vi "2401 Write Data.vi"(7 "I/V":bool, 8 "Compliance":dbl, 10 "Level (A/V)":dbl) -> (1 "Resistance":dbl format="%#_6e", 2 "Current":dbl format="%#_6e", 3 "Voltage":dbl format="%_6e")   [LabVIEW 2011]
panel:
  out "number 4":dbl format="%#_6e"
  out "number5":dbl format="%#_6e"
  out "read buffer":string
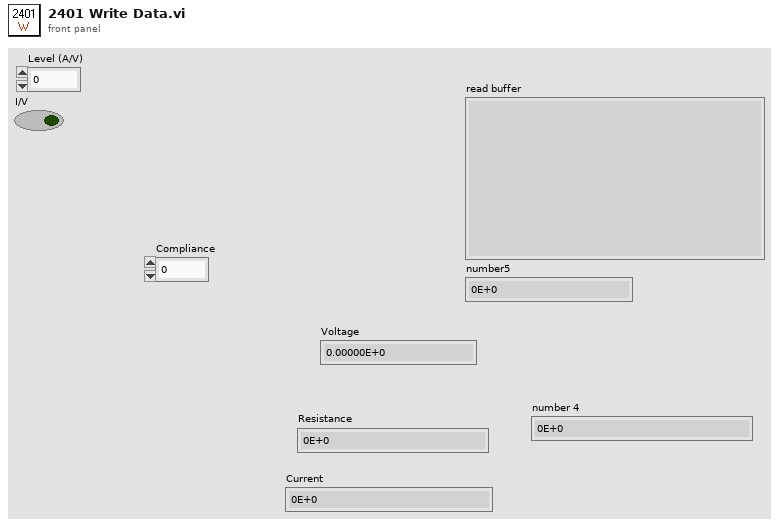
[diagram p1: front panel]
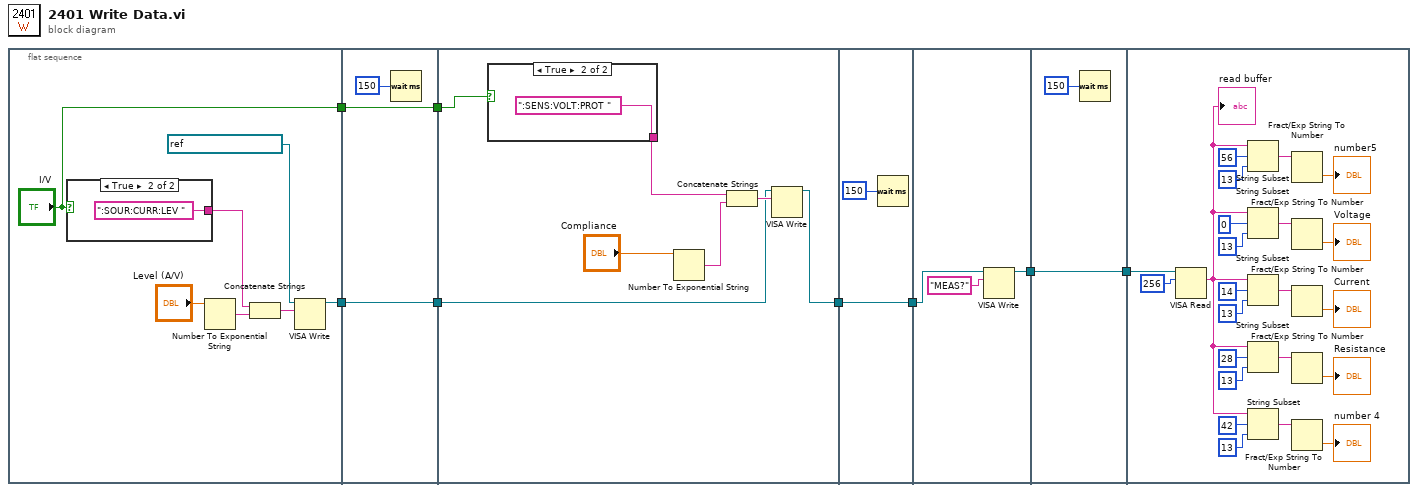
[diagram p0: block diagram]
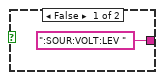
[diagram p2: hidden frame]
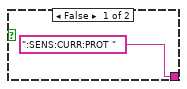
[diagram p3: hidden frame]
diagram:
  n1 = flat-sequence {
    tunnel: [w14] -> w8
    tunnel: ["I/V"] -> w4
    tunnel: w8 -> [w20]
    tunnel: [w20] -> w5
    tunnel: w4 -> [w18]
    tunnel: [w18] -> w3
    tunnel: w5 -> [w23]
    tunnel: [w22] -> w2
    tunnel: w3 -> [w21]
    tunnel: w2 -> [w31]
    tunnel: [w31] -> w1
    tunnel: w1 -> [w33]
    tunnel: [w32] -> w7
    tunnel: w7 -> [w36]
    tunnel: [w36] -> w6
    tunnel: w6 -> [w59]
    frame #0 {
      n2 = case shown="True" "I/V" {
        tunnel: [":SOUR:VOLT:LEV " ("write buffer") ":SOUR:CURR:LEV " ("write buffer")] -> w13
        frame False {
        }
        frame True {
        }
      }
      n3 = Number To Exponential String(number="Level (A/V)") -> (E-format string=w11:string)  [unwired: 3 in]
      n4 = Concatenate Strings(w13, w11) -> (w12:string)
      n5 = VISA Write(VISA resource name=refnum<visa-resource-name> "GPIB0::13::INSTR", write buffer=w12) -> (VISA resource name out=w14:refnum<visa-resource-name>)  [unwired: 1 in, 2 out]
    }
    frame #1 {
      n6 = Wait (ms)(milliseconds to wait=u32 150) -> ()  [unwired: 1 out]
    }
    frame #2 {
      n7 = case shown="True" w21 {
        tunnel: [":SENS:CURR:PROT " ("write buffer") ":SENS:VOLT:PROT " ("write buffer")] -> w27
        frame False {
        }
        frame True {
        }
      }
      n8 = Number To Exponential String(number="Compliance") -> (E-format string=w25:string)  [unwired: 3 in]
      n9 = Concatenate Strings(w27, w25) -> (w26:string)
      n10 = VISA Write(VISA resource name=w23, write buffer=w26) -> (VISA resource name out=w22:refnum<visa-resource-name>)  [unwired: 1 in, 2 out]
    }
    frame #3 {
      n11 = Wait (ms)(milliseconds to wait=u32 150) -> ()  [unwired: 1 out]
    }
    frame #4 {
      n12 = VISA Write(VISA resource name=w33, write buffer="MEAS?") -> (VISA resource name out=w32:refnum<visa-resource-name>)  [unwired: 1 in, 2 out]
    }
    frame #5 {
      n13 = Wait (ms)(milliseconds to wait=u32 150) -> ()  [unwired: 1 out]
    }
    frame #6 {
      n14 = VISA Read(VISA resource name=w59, byte count=u32 256) -> (read buffer=w37:string)  [unwired: 1 in, 3 out]
      "read buffer" <- w37
      n15 = String Subset(string=w37, offset (0)=56, length (rest)=13 ("length (rest)")) -> (substring=w55:string)
      n16 = String Subset(string=w37, offset (0)=0, length (rest)=13 ("length (rest)")) -> (substring=w51:string)
      n17 = String Subset(string=w37, offset (0)=14, length (rest)=13 ("length (rest)")) -> (substring=w47:string)
      n18 = String Subset(string=w37, offset (0)=28, length (rest)=13 ("length (rest)")) -> (substring=w43:string)
      n19 = String Subset(string=w37, offset (0)=42, length (rest)=13 ("length (rest)")) -> (substring=w39:string)
      n20 = Fract/Exp String To Number(string=w55) -> (number=→"number5":dbl)  [unwired: 3 in, 1 out]
      n21 = Fract/Exp String To Number(string=w51) -> (number=→"Voltage":dbl)  [unwired: 3 in, 1 out]
      n22 = Fract/Exp String To Number(string=w47) -> (number=→"Current":dbl)  [unwired: 3 in, 1 out]
      n23 = Fract/Exp String To Number(string=w43) -> (number=→"Resistance":dbl)  [unwired: 3 in, 1 out]
      n24 = Fract/Exp String To Number(string=w39) -> (number=→"number 4":dbl)  [unwired: 3 in, 1 out]
    }
  }
